vi "New Simple Accessor VI Document.vi"(8 "error in":errorcluster, 10 "Write VI":refnum<vi>, 11 "Read VI":refnum<vi>) -> (0 "error out":errorcluster, 2 "Write VI out":refnum<vi>, 3 "Read VI out":refnum<vi>)   [LabVIEW 2014]
doc: "When \"New >> VI For Data Member Access...\" is used to create VIs, this subVI will be invoked if the VIs are created successfully after all other work to create the VIs has been completed. Users may edit this subVI to add any instructions they wish for customizations of the newly generated VIs."
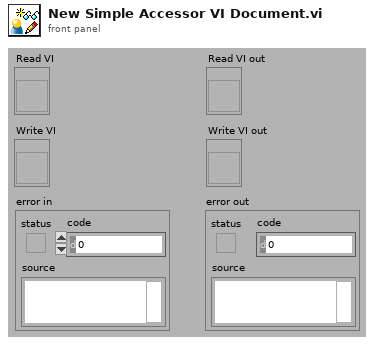
[diagram p1: front panel]
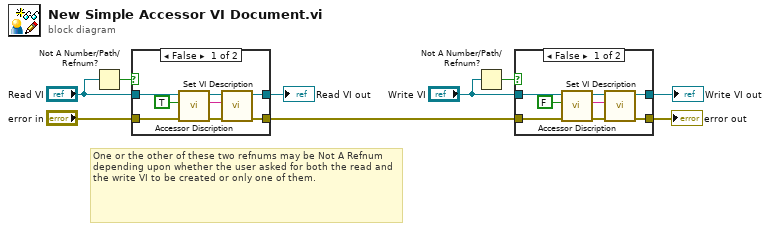
[diagram p0: block diagram]
diagram:
  # "One or the other of these two refnums may be Not A Refnum depending upon whether the user asked for both the read and the write VI to be created or only one of them."
  n1 = Not A Number/Path/Refnum?(number/path/refnum="Read VI") -> (NaN/Path/Refnum?=w8:bool)
  n2 = case shown="False" w8 {
    tunnel: "Read VI" -> [w13 w18]
    tunnel: "error in" -> [w16 w19]
    tunnel: [w17 w19] -> w5
    tunnel: [w10 w18] -> w1
    frame False {
      n3 = call "Accessor Discription.vi"("error in (no error)"=w16, "Read/Write(T->Read)"=TRUE, "VI"=w13) -> ("error out"=w15:errorcluster, "VI Description"=w12:string, "VI out"=w14:refnum<vi>)  [unwired: 6 in]
      n4 = call "Set VI Description.vi"("error in (no error)"=w15, "VI Description"=w12, "VI"=w14) -> ("error out"=w17:errorcluster, "VI out"=w10:refnum<vi>)  [unwired: 7 in]
    }
    frame True {
    }
  }
  "Read VI out" <- w1
  n5 = Not A Number/Path/Refnum?(number/path/refnum="Write VI") -> (NaN/Path/Refnum?=w6:bool)
  n6 = case shown="False" w6 {
    tunnel: "Write VI" -> [w23 w28]
    tunnel: w5 -> [w26 w29]
    tunnel: [w27 w29] -> w3
    tunnel: [w20 w28] -> w2
    frame False {
      n7 = call "Accessor Discription.vi"("error in (no error)"=w26, "Read/Write(T->Read)"=FALSE, "VI"=w23) -> ("error out"=w25:errorcluster, "VI Description"=w22:string, "VI out"=w24:refnum<vi>)  [unwired: 6 in]
      n8 = call "Set VI Description.vi"("error in (no error)"=w25, "VI Description"=w22, "VI"=w24) -> ("error out"=w27:errorcluster, "VI out"=w20:refnum<vi>)  [unwired: 7 in]
    }
    frame True {
    }
  }
  "error out" <- w3
  "Write VI out" <- w2
